vi "Compute Possible Connections.vi"(8 "error in (no error)":errorcluster, 11 "Item Ref in":T2 format="%.0x") -> (0 "error out":errorcluster, 2 "Possible Connections":T1[](array[typedef]), 3 "Item Ref out":T2 format="%.0x")   [LabVIEW 2017, in "SLSC Switch Scripting.lvlib"]
uses:
  SLSC Switch Scripting.lvlib
  <vilib>/NI Veristand/Custom Device API/Custom Device Item Ref.ctl
  Shared/Routing and Faulting Hardware API/Types/Possible Connections for Endpoint.ctl
  <vilib>/SLSC_Switch/Path Capability.ctl
  <vilib>/SLSC_Switch/Initialize with Topology (Simulate).vi
  <vilib>/SLSC_Switch/SLSC Switch.lvlib
  <resource>/objmgr/nislscsl.rc
  Shared/Routing and Faulting Hardware API/Routing and Faulting Hardware API.lvlib
  <vilib>/NI Veristand/Custom Device API/Custom Device API.lvlib
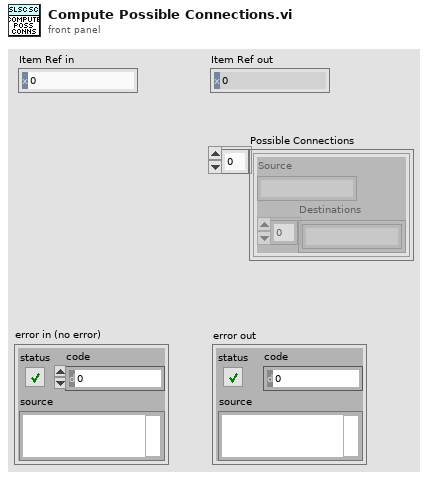
[diagram p1: front panel]
types:
  T1 = typedef "Routing and Faulting Hardware API.lvlib/Possible Connections for Endpoint.ctl" = cluster{"Source":string, "Destinations":string[]}
  T2 = typedef "Custom Device API.lvlib/Custom Device Item Ref.ctl" = u64
  T3 = typedef "nislscslSession.ctl" = refnum<k20>
  T4 = typedef "SLSC Switch Shared.lvlib/Endpoint Configuration Enum.ctl" = enum16{"Load", "Source", "Configuration"}
  T5 = typedef "SLSC Switch.lvlib/Path Capability.ctl" = i32
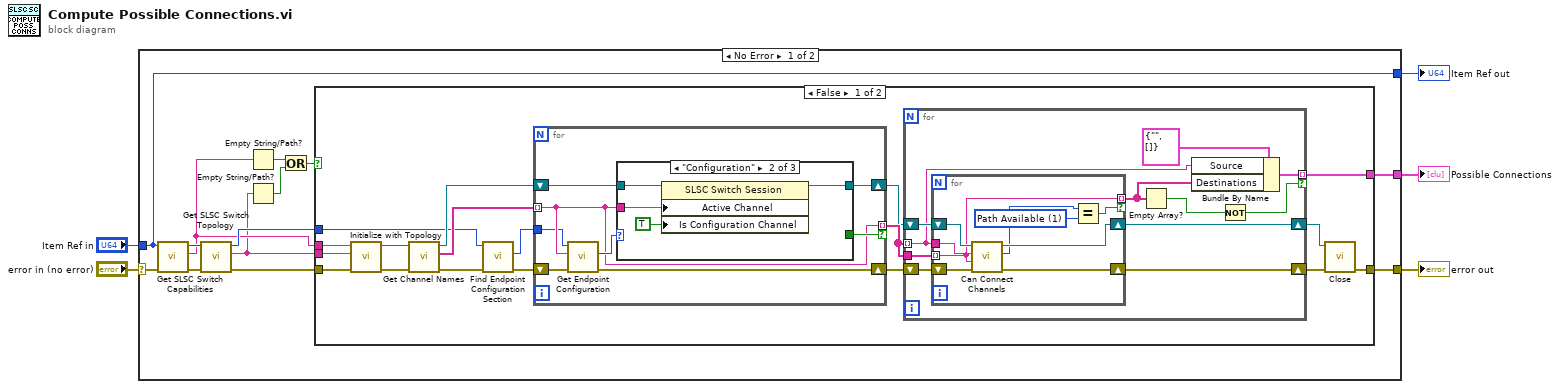
[diagram p0: block diagram]
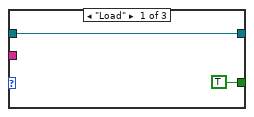
[diagram p2: hidden frame]
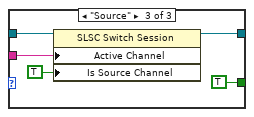
[diagram p3: hidden frame]
diagram:
  n1 = case shown="No Error" "error in (no error)" {
    selector: "error in (no error)" -> [w14 w78]
    tunnel: [w18 w78] -> w5
    tunnel: "Item Ref in" -> [w8 w77]
    tunnel: [w8 w77] -> w3
    tunnel: [w12 _] -> w1
    frame No Error {
      n2 = call "Get SLSC Switch Capabilities.vi"("error in (no error)"=w14, "SLSC Switch Custom Device Ref in"=w8) -> ("error out"=w17:errorcluster, "Capabilities"=w11:string, "SLSC Switch Custom Device Ref out"=w16:T2)  [unwired: 7 in]
      n3 = call "Get SLSC Switch Topology.vi"("error in (no error)"=w17, "SLSC Switch Custom Device Ref in"=w16) -> ("error out"=w13:errorcluster, "Topology"=w10:string, "SLSC Switch Custom Device Ref out"=w15:T2)  [unwired: 7 in]
      n4 = Empty String/Path?(string/path=w11) -> (empty?=w6:bool)
      n5 = Empty String/Path?(string/path=w10) -> (empty?=w7:bool)
      n6 = Or(x=w6, y=w7) -> (x .or. y?=w9:bool)
      n7 = case shown="False" w9 {
        tunnel: [w27 w76] -> w18
        tunnel: w11 -> [w26 _]
        tunnel: w10 -> [w25 _]
        tunnel: w15 -> [w20 _]
        tunnel: w13 -> [w24 w76]
        tunnel: [w23 _] -> w12
        frame False {
          n8 = call-poly <vilib>:"Initialize with Topology.vi"("error in (no error)"=w24, "topology"=w25, "switches json"=w26) -> ("error out"=w32:errorcluster, "session out"=w35:T3)  [unwired: 7 in]
          n9 = call <vilib>:"Get Channel Names.vi"("error in (no error)"=w32, "session in"=w35) -> ("error out"=w22:errorcluster, "channel names"=w33:string[], "session out"=w34:T3)  [unwired: 7 in]
          n10 = call "Find Endpoint Configuration Section.vi"("error in (no error)"=w22, "SLSC Switch Custom Device Ref in"=w20) -> ("error out"=w21:errorcluster, "Endpoint Config Section Ref"=w19:T2)  [unwired: 7 in, 1 out]
          n11 = for {
            tunnel: [w61] -> w36 mode=indexing if=w63
            tunnel: w33 -> [w61] mode=indexing
            tunnel: w19 -> [w60]
            shift-right: [w58] -> w31
            shift-left: w21 -> [w59]
            shift-right: [w57] -> w30
            shift-left: w34 -> [w64]
            n12 = call "Get Endpoint Configuration.vi"("error in (no error)"=w59, "Endpoint"=w61, "Endpoint Configuration Section Ref in"=w60) -> ("error out"=w58:errorcluster, "Configuration Type"=w62:T4)  [unwired: 6 in, 1 out]
            n13 = case shown="\"Configuration\"" w62 {
              tunnel: w64 -> [w65 w69 w75]
              tunnel: w61 -> [_ w70 w73]
              tunnel: [TRUE _ TRUE] -> w63
              tunnel: [w65 w67 w71] -> w57
              frame "Load" {
              }
              frame "Configuration" {
                n14 = property class="SLSC Switch Session"(reference=w69, "Active Channel"=w70, "Is Configuration Channel"=TRUE ("Channel Configuration:Is Configuration Channel")) -> (reference out=w67:T3)  [unwired: 1 in, 1 out]
              }
              frame "Source" {
                n15 = property class="SLSC Switch Session"(reference=w75, "Active Channel"=w73, "Is Source Channel"=TRUE ("Channel Configuration:Is Source Channel")) -> (reference out=w71:T3)  [unwired: 1 in, 1 out]
              }
            }
          }
          n16 = for {
            tunnel: w36 -> [w41] mode=indexing
            tunnel: w36 -> [w47]
            shift-right: [w45] -> w29
            shift-left: w31 -> [w46]
            shift-right: [w43] -> w28
            shift-left: w30 -> [w44]
            tunnel: [w38] -> w23 mode=indexing if=w37
            n17 = for {
              tunnel: w47 -> [w49] mode=indexing
              shift-right: [w55] -> w45
              shift-left: w46 -> [w56]
              shift-right: [w53] -> w43
              shift-left: w44 -> [w54]
              tunnel: w41 -> [w52]
              tunnel: [w49] -> w39 mode=indexing if=w48
              w50 = T5 1 items=["Path Available"=1, "Path Exists"=2, "Path Unsupported"=3, "Resource in Use"=4, "Source Conflict"=5, "Channel Not Available"=6] ("y")
              n18 = call <vilib>:"Can Connect Channels.vi"("error in (no error)"=w56, "channel 2"=w49, "channel 1"=w52, "session in"=w54) -> ("error out"=w55:errorcluster, "path capability"=w51:T5, "session out"=w53:T3)  [unwired: 5 in]
              n19 = Equal?(x=w51, y=w50) -> (x = y?=w48:bool)
            }
            n20 = Empty Array?(array=w39) -> (empty?=w40:bool)
            n21 = Bundle By Name(cluster=T1 {"Source"="", "Destinations"=[]} ("Possible Connections for Endpoint"), "Source"=w41, "Destinations"=w39) -> (w38:T1)
            n22 = Not(x=w40) -> (.not. x?=w37:bool)
          }
          n23 = call <vilib>:"Close.vi"("error in (no error)"=w29, "session in"=w28) -> ("error out"=w27:errorcluster)  [unwired: 9 in]
        }
        frame True {
        }
      }
    }
    frame Error {
    }
  }
  "error out" <- w5
  "Item Ref out" <- w3
  "Possible Connections" <- w1
